vi "ProdaNG.Convert.String-U8[].vi"(0 "Input String":string, 1 "Size":i32) -> (2 "Output":u8[](array[numeric]))   [LabVIEW 2016]
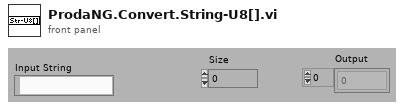
[diagram p1: front panel]
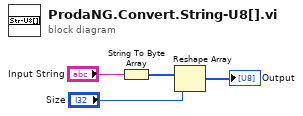
[diagram p0: block diagram]
diagram:
  n1 = String To Byte Array(string="Input String") -> (unsigned byte array=w4:u8[])
  n2 = Reshape Array(w4, "Size") -> (→"Output":u8[])
